vi "Omron Serial FINS-Read Data(I16 Array).vi"(8 "error in":errorcluster, 10 "Read Setting(I16 Array)":T1={"I/O Memory Address"=130, "Beginning Address"=0, "No. Of Items"=0} {"I/O Memory Address" items=["DM"=130, "CIO"=176, "WR"=177, "HR"=178, "AR"=179, "TIM"=137, "EM"=152]}, 11 "Buffer Data In":T2={"VISA Resource Name"="", "Wait For Read(ms)"=50, "Command Code"=enum."Memory area read", "Command String"="", "Read Bytes"=0, "Response String"=""}) -> (0 "error out":errorcluster, 2 "Data":i16[](array[numeric]), 3 "Buffer Data Out":T2={"VISA Resource Name"="", "Wait For Read(ms)"=50, "Command Code"=enum."Memory area read", "Command String"="", "Read Bytes"=0, "Response String"=""})   [LabVIEW 2016]
uses:
  Data Def/Omron Serial FINS-Buffer Data.ctl
  Data Def/Omron Serial FINS-Command Code.ctl
  Data Def/Omron Serial FINS-FINS Command Frame.ctl
  Data Def/Omron Serial FINS-Memory Area Read Data.ctl
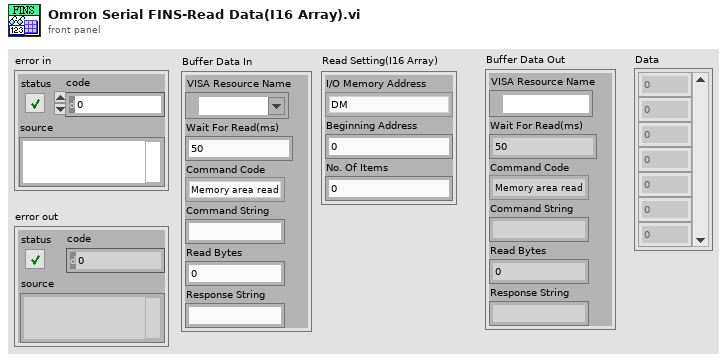
[diagram p1: front panel]
types:
  T1 = cluster{"I/O Memory Address":i32, "Beginning Address":u32, "No. Of Items":u32}
  T2 = typedef "Omron Serial FINS-Buffer Data.ctl" = cluster{"VISA Resource Name":refnum<visa-resource-name>, "Wait For Read(ms)":u32, "Command Code":T3, "Command String":string, "Read Bytes":u32, "Response String":string}
  T3 = typedef "Omron Serial FINS-Command Code.ctl" = enum16{"Memory area read", "Memory area write"}
  T4 = typedef "Omron Serial FINS-Memory Area Read Data.ctl" = cluster{"I/O Memory Address":i32, "Beginning Address":u32, "No. Of Items":u32}
  T5 = typedef "Omron Serial FINS-FINS Command Frame.ctl" = cluster{"Unit Number":u8, "Response Wait Time":u8, "Command Code":T3, "Command Data":variant}
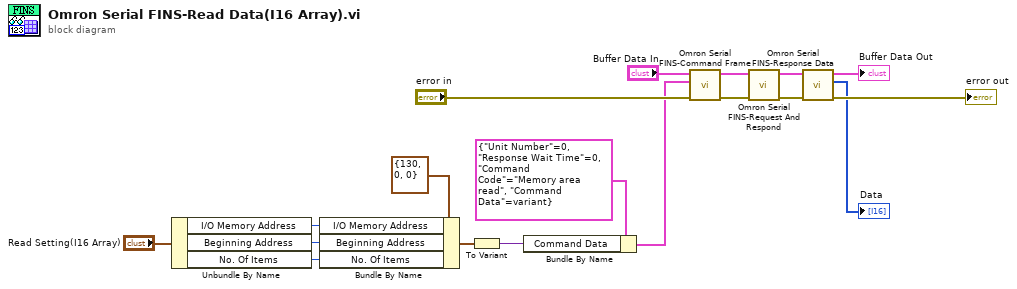
[diagram p0: block diagram]
diagram:
  n1 = Unbundle By Name("Read Setting(I16 Array)") -> ("I/O Memory Address"=w3:i32, "Beginning Address"=w2:u32, "No. Of Items"=w1:u32)
  n2 = Bundle By Name(cluster=T4 {"I/O Memory Address"=130, "Beginning Address"=0, "No. Of Items"=0} ("Memory Area Read Data"), "I/O Memory Address"=w3, "Beginning Address"=w2, "No. Of Items"=w1) -> (w5:T4)
  n3 = To Variant(anything=w5) -> (Variant=w16:variant)
  n4 = Bundle By Name(cluster=T5 {"Unit Number"=0, "Response Wait Time"=0, "Command Code"=enum."Memory area read", "Command Data"=variant} ("FINS Command Frame"), "Command Data"=w16) -> (w14:T5)
  n5 = call "Omron Serial FINS-Command Frame.vi"("error in"="error in", "FINS Command Frame"=w14, "Buffer Data In"="Buffer Data In") -> ("error out"=w12:errorcluster, "Buffer Data Out"=w13:T2)  [unwired: 7 in]
  n6 = call "Omron Serial FINS-Request And Respond.vi"("error in"=w12, "Buffer Data In"=w13) -> ("error out"=w10:errorcluster, "Buffer Data Out"=w11:T2)  [unwired: 8 in]
  n7 = call "Omron Serial FINS-Response Data.vi"("error in"=w10, "Buffer Data In"=w11) -> ("error out"=→"error out":errorcluster, "Data"=→"Data":i16[], "Buffer Data Out"=→"Buffer Data Out":T2)  [unwired: 7 in]
